vi "Set piezo voltage.vi"(0 "Piezo handle":i32, 5 "X Voltage":dbl min=0.0 max=100.0, 7 "Y Voltage":dbl min=0.0 max=100.0, 9 "Z Voltage":dbl min=0.0 max=100.0, 11 "Piezo error in":errorcluster) -> (4 "Piezo handle out":i32, 15 "Piezo error out":errorcluster)   [LabVIEW 2017]
uses:
  <instrlib>/Thorlabs_MDT69xB/Thorlabs_MDT69xB.lvlib
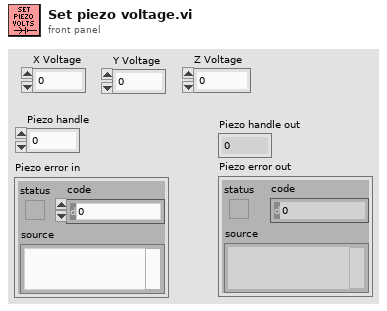
[diagram p1: front panel]
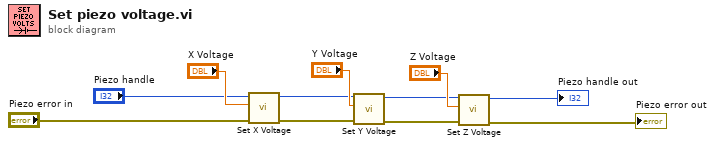
[diagram p0: block diagram]
diagram:
  n1 = call <instrlib>:"Set X Voltage.vi"("error in (no error)"="Piezo error in", "x Voltage"="X Voltage", "hdl in"="Piezo handle") -> ("error out"=w6:errorcluster, "hdl"=w5:i32)  [unwired: 7 in]
  n2 = call <instrlib>:"Set Y Voltage.vi"("error in (no error)"=w6, "Y Voltage"="Y Voltage", "hdl in"=w5) -> ("error out"=w3:errorcluster, "hdl"=w4:i32)  [unwired: 7 in]
  n3 = call <instrlib>:"Set Z Voltage.vi"("error in (no error)"=w3, "z Voltage"="Z Voltage", "hdl in"=w4) -> ("error out"=→"Piezo error out":errorcluster, "hdl"=→"Piezo handle out":i32)  [unwired: 7 in]
